vi "Test SD 2.vi"() -> ()   [LabVIEW 2014]
uses:
  LabVIEW Universal Transcriptor SD Card Library.lvlib
  <vilib>/LabVIEW Universal Transcriptor/LabVIEW to Arduino Transcriptor/Transcriptors/System API/System Serial Library Variables/System Serial Library Variables.lvlib
  <vilib>/LabVIEW Universal Transcriptor/LabVIEW to Arduino Transcriptor/Transcriptors/System API/Serial println string.vi
  File Class/write float.vi
  File Class/write bytes.vi
  File.lvclass
panel:
  out "String Buffer":string
  out "error out":errorcluster
  in  "Error In":errorcluster
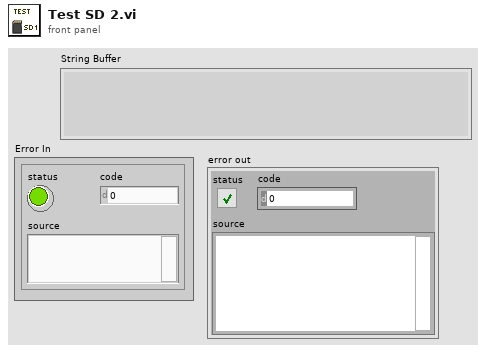
[diagram p1: front panel]
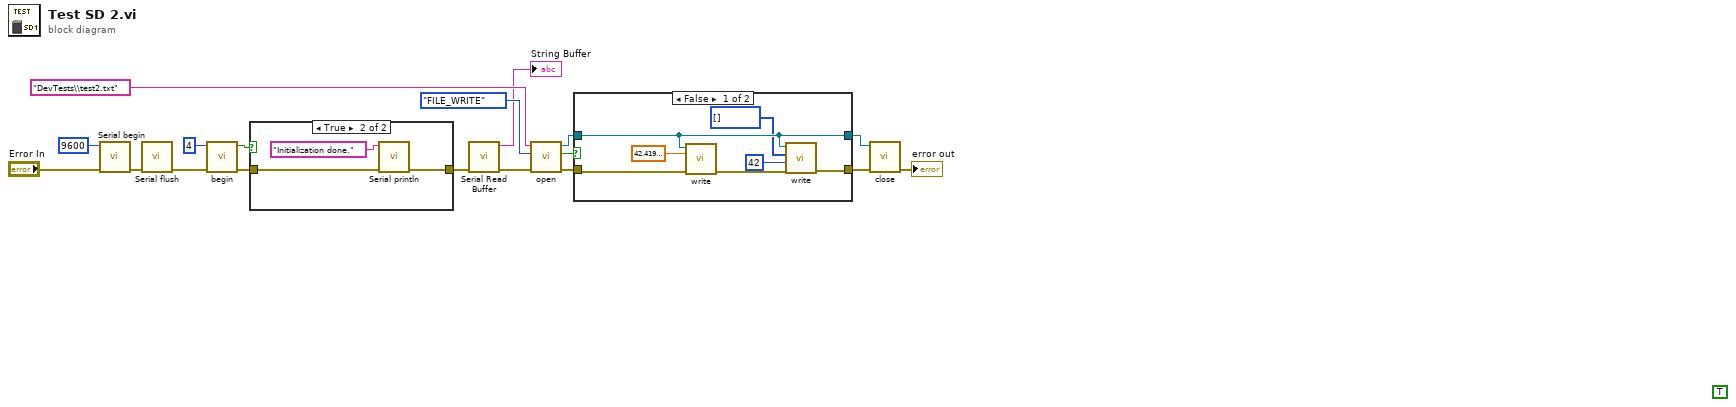
[diagram p0: block diagram]
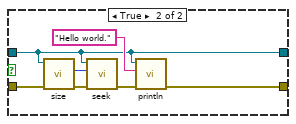
[diagram p2: hidden frame]
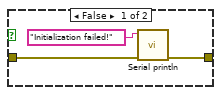
[diagram p3: hidden frame]
diagram:
  (unwired) TRUE
  n1 = call <vilib>:"Serial begin.vi"("Error In"="Error In", "speed (Bd)"=9600) -> ("Error Out"=w4:errorcluster)  [unwired: 9 in]
  n2 = call <vilib>:"Serial flush.vi"("Error In"=w4) -> ("Error Out"=w3:errorcluster)  [unwired: 10 in]
  n3 = call "begin.vi"("Error In"=w3, "CS pin (optional)"=u8 4) -> ("Error Out"=w15:errorcluster, "success?"=w14:bool)  [unwired: 8 in]
  n4 = case shown="True" w14 {
    tunnel: w15 -> [w20 w23]
    tunnel: [w19 w22] -> w6
    frame False {
      n5 = call-poly <vilib>:"Serial println.vi"("Error In"=w20, "string in"="Initialization failed!" ("filepath")) -> ("Error Out"=w19:errorcluster)  [unwired: 9 in]
    }
    frame True {
      n6 = call-poly <vilib>:"Serial println.vi"("Error In"=w23, "string in"="Initialization done." ("filepath")) -> ("Error Out"=w22:errorcluster)  [unwired: 9 in]
    }
  }
  n7 = call <vilib>:"Serial Read Buffer.vi"("Error In"=w6) -> ("Error Out"=w2:errorcluster, "String Buffer"=→"String Buffer":string)  [unwired: 9 in]
  n8 = call "open.vi"("Error In"=w2, "mode"=enum16{"FILE_READ", "FILE_WRITE"}."FILE_WRITE", "filepath"="DevTests\\test2.txt") -> ("Error Out"=w10:errorcluster, "opened?"=w9:bool, "File out"=w11:refnum<class "File.lvclass">)  [unwired: 6 in]
  n9 = case shown="False" w9 {
    tunnel: w11 -> [w27 w32]
    tunnel: w10 -> [w31 w33]
    tunnel: [w29 w38] -> w8
    tunnel: [w27 w32] -> w7
    frame False {
      n10 = call-poly "write.vi"("error in (no error)"=w31, "number"=sgl 42.42, "File in"=w27) -> ("error out"=w28:errorcluster)  [unwired: 8 in]
      n11 = call-poly "write.vi"("error in (no error)"=w28, "length"=u32 42, "buffer"=u8[] [], "File in"=w27) -> ("error out"=w29:errorcluster)  [unwired: 7 in]
    }
    frame True {
      n12 = call-dynamic "size.vi"("error in (no error)"=w33, "File in"=w32) -> ("error out"=w37:errorcluster, "size"=w34:u32)  [unwired: 7 in]
      n13 = call-dynamic "seek.vi"("error in (no error)"=w37, "position"=w34, "File in"=w32) -> ("error out"=w36:errorcluster)  [unwired: 8 in]
      n14 = call-dynamic "println.vi"("error in (no error)"=w36, "String"="Hello world.", "File in"=w32) -> ("error out"=w38:errorcluster)  [unwired: 8 in]
    }
  }
  n15 = call-dynamic "close.vi"("error in (no error)"=w8, "File in"=w7) -> ("error out"=→"error out":errorcluster)  [unwired: 9 in]
